vi "Vision - Get ThumbNail Dimensions.vi"(7 "Device Type":T2, 8 "error in (no error)":errorcluster, 11 "# of Images":dbl) -> (0 "error out":errorcluster, 3 "ThumbNail Dims":T1)   [LabVIEW 2024]
uses:
  Controls/Device_Type.ctl
  Controls/ThumbNail Dimensions.ctl
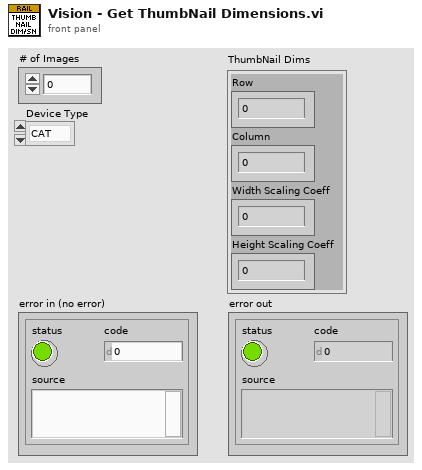
[diagram p1: front panel]
types:
  T1 = typedef "ThumbNail Dimensions.ctl" = cluster{"Row":i32, "Column":i32, "Width Scaling Coeff":dbl, "Height Scaling Coeff":dbl}
  T2 = typedef "Device_Type.ctl" = enum16{"CAT", "Bi-CAT", "YRCA", "RCA", "RV-HR", "TV-HR"}
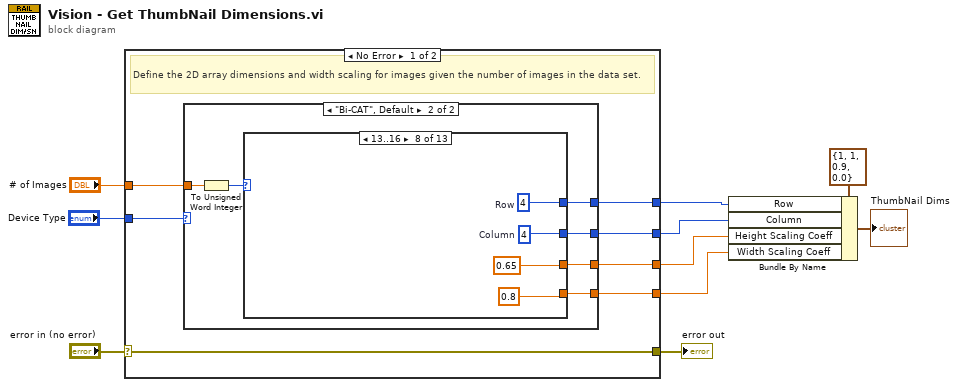
[diagram p0: block diagram]
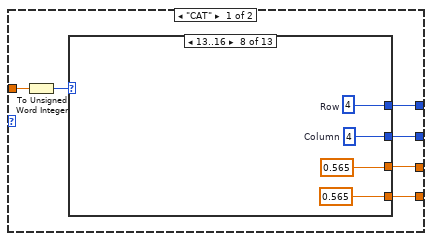
[diagram p2: hidden frame]
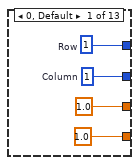
[diagram p3: hidden frame]
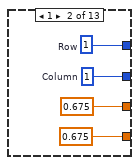
[diagram p4: hidden frame]
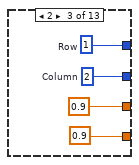
[diagram p5: hidden frame]
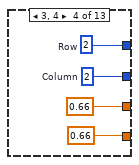
[diagram p6: hidden frame]
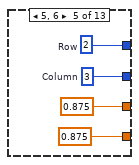
[diagram p7: hidden frame]
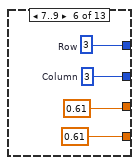
[diagram p8: hidden frame]
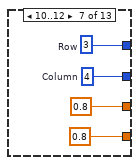
[diagram p9: hidden frame]
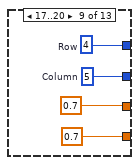
[diagram p10: hidden frame]
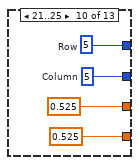
[diagram p11: hidden frame]
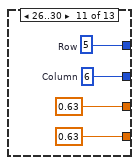
[diagram p12: hidden frame]
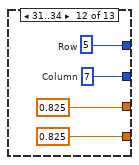
[diagram p13: hidden frame]
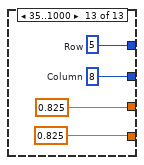
[diagram p14: hidden frame]
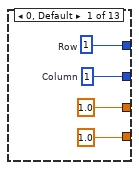
[diagram p15: hidden frame]
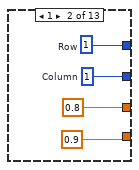
[diagram p16: hidden frame]
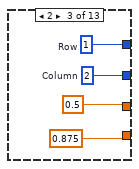
[diagram p17: hidden frame]
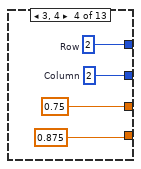
[diagram p18: hidden frame]
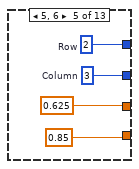
[diagram p19: hidden frame]
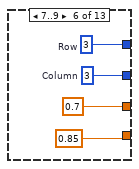
[diagram p20: hidden frame]
diagram:
  n1 = case shown="No Error" "error in (no error)" {
    selector: "error in (no error)" -> [w14 w136]
    tunnel: [w13 w134] -> w1
    tunnel: [w17 w135] -> w3
    tunnel: [w16 w135] -> w4
    tunnel: "# of Images" -> [w15 _]
    tunnel: [w14 w136] -> w9
    tunnel: "Device Type" -> [w12 _]
    tunnel: [w11 w134] -> w2
    frame No Error {
      # "Define the 2D array dimensions and width scaling for images given the number of images in the data set."
      n2 = case shown="\"Bi-CAT\", Default" w12 {
        tunnel: [w23 w81] -> w17
        tunnel: [w22 w80] -> w16
        tunnel: w15 -> [w20 w78]
        tunnel: [w19 w77] -> w13
        tunnel: [w18 w76] -> w11
        frame "CAT" {
          n3 = To Unsigned Word Integer(number=w20) -> (unsigned 16bit integer=w21:u16)
          n4 = case shown="13..16" w21 {
            tunnel: [w27 w31 w35 w39 w43 w47 w51 w55 w59 w63 w67 w71 w75] -> w22
            tunnel: [w26 w30 w34 w38 w42 w46 w50 w54 w58 w62 w66 w70 w74] -> w23
            tunnel: [1.0 ("x") 0.675 ("x") 0.9 ("x") 0.66 ("x") 0.875 ("x") 0.61 ("x") 0.8 ("x") 0.565 ("x") 0.7 ("x") 0.525 ("x") 0.63 ("x") 0.825 ("x") 0.825 ("x")] -> w19
            tunnel: [1.0 ("x") 0.675 ("x") 0.9 ("x") 0.66 ("x") 0.875 ("x") 0.61 ("x") 0.8 ("x") 0.565 ("x") 0.7 ("x") 0.525 ("x") 0.63 ("x") 0.825 ("x") 0.825 ("x")] -> w18
            frame 0, Default {
              w26 = 1  # Column
              w27 = 1  # Row
            }
            frame 1 {
              w30 = 1  # Column
              w31 = 1  # Row
            }
            frame 2 {
              w34 = 2  # Column
              w35 = 1  # Row
            }
            frame 3, 4 {
              w38 = 2  # Column
              w39 = 2  # Row
            }
            frame 5, 6 {
              w42 = 3  # Column
              w43 = 2  # Row
            }
            frame 7..9 {
              w46 = 3  # Column
              w47 = 3  # Row
            }
            frame 10..12 {
              w50 = 4  # Column
              w51 = 3  # Row
            }
            frame 13..16 {
              w54 = 4  # Column
              w55 = 4  # Row
            }
            frame 17..20 {
              w58 = 5  # Column
              w59 = 4  # Row
            }
            frame 21..25 {
              w62 = 5  # Column
              w63 = 5  # Row
            }
            frame 26..30 {
              w66 = 6  # Column
              w67 = 5  # Row
            }
            frame 31..34 {
              w70 = 7  # Column
              w71 = 5  # Row
            }
            frame 35..1000 {
              w74 = 8  # Column
              w75 = 5  # Row
            }
          }
        }
        frame "Bi-CAT", Default {
          n5 = To Unsigned Word Integer(number=w78) -> (unsigned 16bit integer=w79:u16)
          n6 = case shown="13..16" w79 {
            tunnel: [w85 w89 w93 w97 w101 w105 w109 w113 w117 w121 w125 w129 w133] -> w80
            tunnel: [w84 w88 w91 w96 w100 w104 w108 w112 w116 w120 w124 w128 w132] -> w81
            tunnel: [1.0 ("x") 0.9 ("x") 0.875 ("x") 0.875 ("x") 0.85 ("x") 0.85 ("x") 0.825 ("x") 0.8 ("x") 0.8 ("x") 0.73 ("x") 0.775 ("x") 0.75 ("x") 0.725 ("x")] -> w77
            tunnel: [1.0 ("x") 0.8 ("x") 0.5 ("x") 0.75 ("x") 0.625 ("x") 0.7 ("x") 0.68 ("x") 0.65 ("x") 0.63 ("x") 0.58 ("x") 0.58 ("x") 0.6 ("x") 0.525 ("x")] -> w76
            frame 0, Default {
              w84 = 1  # Column
              w85 = 1  # Row
            }
            frame 1 {
              w88 = 1  # Column
              w89 = 1  # Row
            }
            frame 2 {
              w91 = 2  # Column
              w93 = 1  # Row
            }
            frame 3, 4 {
              w96 = 2  # Column
              w97 = 2  # Row
            }
            frame 5, 6 {
              w100 = 3  # Column
              w101 = 2  # Row
            }
            frame 7..9 {
              w104 = 3  # Column
              w105 = 3  # Row
            }
            frame 10..12 {
              w108 = 4  # Column
              w109 = 3  # Row
            }
            frame 13..16 {
              w112 = 4  # Column
              w113 = 4  # Row
            }
            frame 17..20 {
              w116 = 5  # Column
              w117 = 4  # Row
            }
            frame 21..25 {
              w120 = 5  # Column
              w121 = 5  # Row
            }
            frame 26..30 {
              w124 = 6  # Column
              w125 = 5  # Row
            }
            frame 31..34 {
              w128 = 7  # Column
              w129 = 5  # Row
            }
            frame 35..1000 {
              w132 = 8  # Column
              w133 = 5  # Row
            }
          }
        }
      }
    }
    frame Error {
      w134 = 1.0 ("x")
      w135 = 1 ("Row")
    }
  }
  "error out" <- w9
  n7 = Bundle By Name(cluster=T1 {"Row"=1, "Column"=1, "Width Scaling Coeff"=0.9, "Height Scaling Coeff"=0.0} ("Cluster"), "Row"=w4, "Column"=w3, "Height Scaling Coeff"=w2, "Width Scaling Coeff"=w1) -> (→"ThumbNail Dims":T1)
